vi "Evaluate.vi"(8 "error in (no error)":errorcluster, 11 "One or More In":refnum<class "One or More.lvclass">) -> (0 "error out":errorcluster, 1 "Message":string, 2 "Passed?":bool)   [LabVIEW 2020, in "One or More.lvlib" / "One or More.lvclass"]
uses:
  One or More.lvclass
  One or More.lvclass/One or More.ctl
  Core/VI Call/VI Call.lvclass
  Core/Comparator/Comparator.lvclass
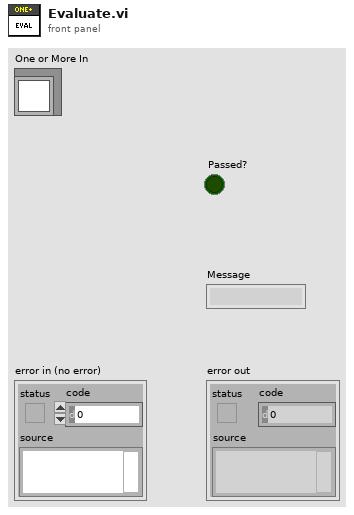
[diagram p1: front panel]
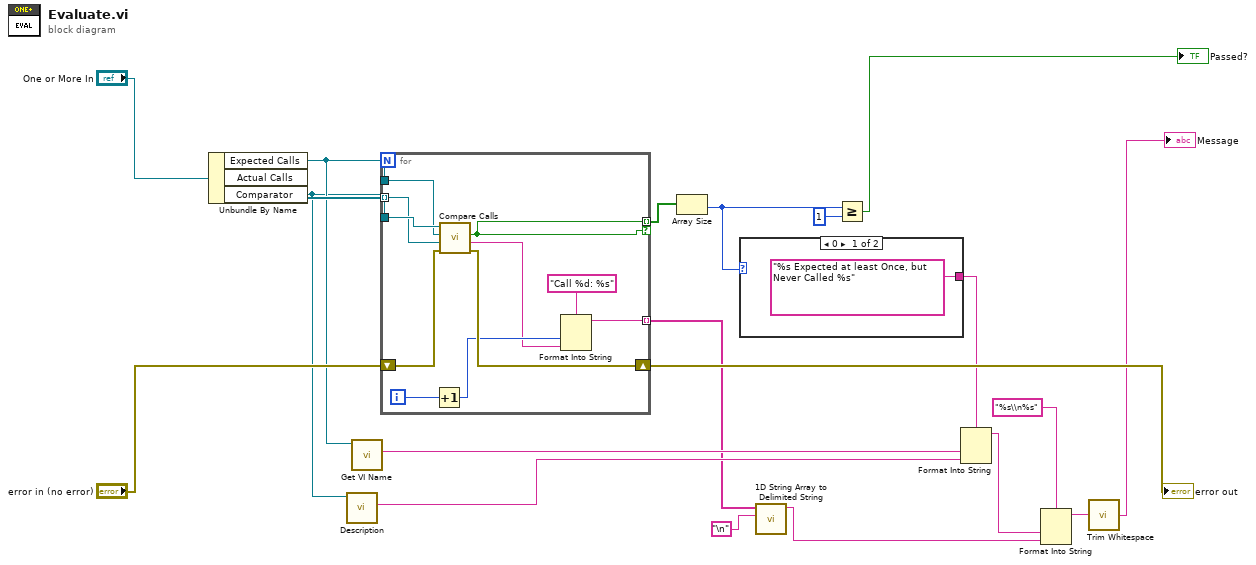
[diagram p0: block diagram]
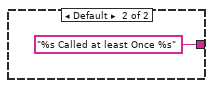
[diagram p2: hidden frame]
diagram:
  n1 = Unbundle By Name("One or More In") -> ("Expected Calls"=w11:refnum<class "VI Call.lvclass">, "Actual Calls"=w17:refnum<class "VI Call.lvclass">[], "Comparator"=w10:refnum<class "Comparator.lvclass">)
  n2 = call-dynamic "Description.vi"("Comparator in"=w10) -> ("Description"=w13:string)  [unwired: 9 in, 1 out]
  n3 = call-dynamic "Get VI Name.vi"("VI Call In"=w11) -> ("VI Name"=w12:string)  [unwired: 9 in, 1 out]
  n4 = for {
    tunnel: w11 -> [w30]
    tunnel: w10 -> [w31]
    tunnel: w17 -> [w29] mode=indexing
    shift-right: [w27] -> w15
    shift-left: "error in (no error)" -> [w28]
    tunnel: [w26] -> w19 mode=indexing if=w26
    tunnel: [w21] -> w3 mode=indexing
    i -> [w24]
    n5 = Increment(x=w24) -> (x+1=w23:i32)
    n6 = call-dynamic "Compare Calls.vi"("error in (no error)"=w28, "VI Call 2"=w29, "VI Call 1"=w30, "Comparator in"=w31) -> ("error out"=w27:errorcluster, "Description"=w22:string, "Equal?"=w26:bool)  [unwired: 5 in]
    n7 = Format Into String(format string="Call %d: %s", w23, w22) -> (resulting string=w21:string)  [unwired: 2 in, 1 out]
  }
  "error out" <- w15
  n8 = Array Size(array=w19) -> (size(s)=w9:i32)
  n9 = case shown="0" w9 {
    tunnel: ["%s Expected at least Once, but Never Called %s" ("Message") "%s Called at least Once %s" ("Message")] -> w8
    frame 0 {
    }
    frame Default {
    }
  }
  n10 = call <vilib>:"1D String Array to Delimited String.vi"("delimiter"="\n", "string array"=w3) -> ("delimited string"=w2:string)  [unwired: 9 in]
  n11 = Greater Or Equal?(x=w9, y=1) -> (x >= y?=→"Passed?":bool)
  n12 = Format Into String(format string=w8, w12, w13) -> (resulting string=w1:string)  [unwired: 2 in, 1 out]
  n13 = Format Into String(format string="%s\\n%s", w1, w2) -> (resulting string=w6:string)  [unwired: 2 in, 1 out]
  n14 = call <vilib>:"Trim Whitespace.vi"("string"=w6) -> ("trimmed string"=→"Message":string)  [unwired: 1 in]
